vi "Create Example PNG.vi"() -> ()   [LabVIEW 2017]
panel:
  out "path":path
  in  "Error In":errorcluster
  out "Error Out":errorcluster
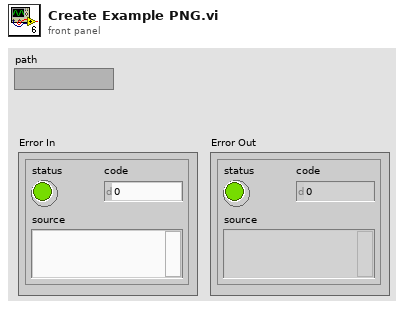
[diagram p1: front panel]
types:
  T1 = typedef "imagedata.ctl" = cluster{"image type":i32, "image depth":i32, "image":u8[], "mask":u8[], "colors":u32[], "Rectangle":cluster{"left":i16, "top":i16, "right":i16, "bottom":i16}}
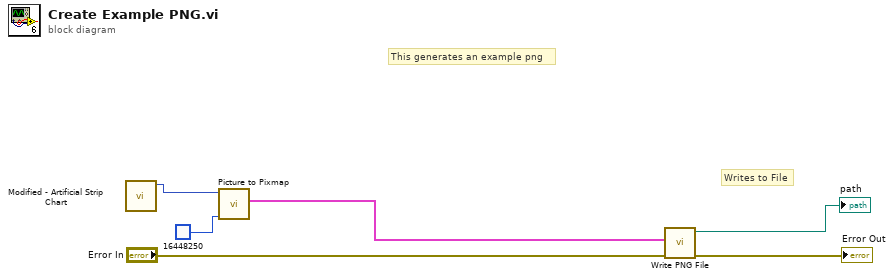
[diagram p0: block diagram]
diagram:
  # "This generates an example png"
  # "Writes to File"
  n1 = call "Modified - Artificial Strip Chart.vi"() -> ("Output 2D Image"=w6:picture)  [unwired: 11 in]
  n2 = call <vilib>:"Picture to Pixmap.vi"("Background Color"=u32 16448250, "picture"=w6) -> ("image data"=w5:T1)  [unwired: 8 in, 1 out]
  n3 = call <vilib>:"Write PNG File.vi"("error in (no error)"="Error In", "image data"=w5) -> ("error out"=→"Error Out":errorcluster, "path"=→"path":path)  [unwired: 8 in]
